vi "__2400_init.vi"(4 "‚SW":bool=TRUE, 5 "volt_range(mV)":dbl, 6 "curr_range(mA)":dbl, 7 "GPIB":string="24") -> (0 "error out":errorcluster caption="エラー出力")   [LabVIEW 2017]
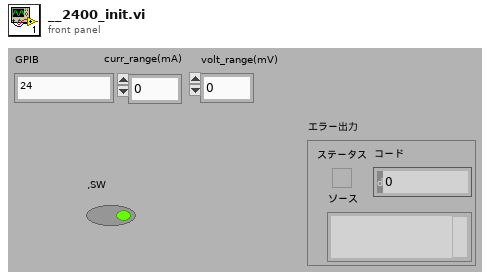
[diagram p1: front panel]
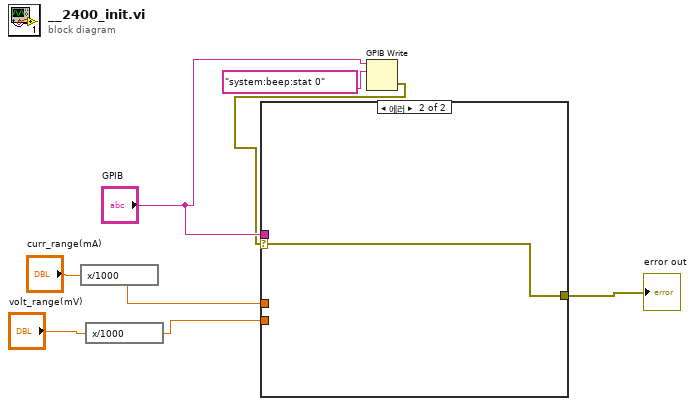
[diagram p0: block diagram]
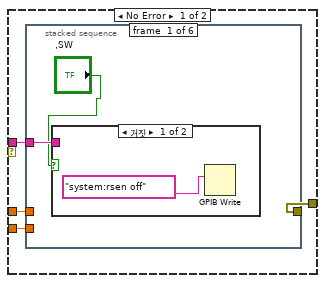
[diagram p2: hidden frame]
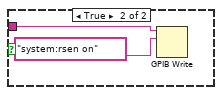
[diagram p3: hidden frame]
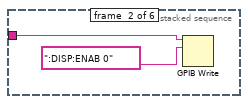
[diagram p4: hidden frame]
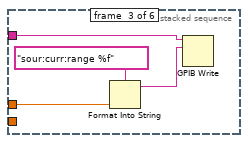
[diagram p5: hidden frame]
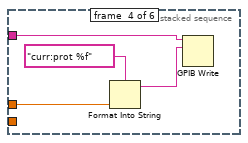
[diagram p6: hidden frame]
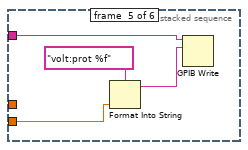
[diagram p7: hidden frame]
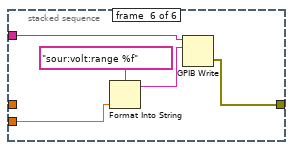
[diagram p8: hidden frame]
diagram:
  n1 = expression code="x/1000"("curr_range(mA)") -> (w7:dbl)
  n2 = expression code="x/1000"("volt_range(mV)") -> (w5:dbl)
  n3 = GPIB Write(0:"GPIB", 1:"system:beep:stat 0") -> (6:w1:errorcluster)  [unwired: 3 in, 1 out]
  n4 = case shown="에러" w1 {
    selector: w1 -> [_ w37]
    tunnel: w7 -> [w12 _]
    tunnel: w5 -> [w11 _]
    tunnel: [w10 w37] -> w4
    tunnel: "GPIB" -> [w9 _]
    frame No Error {
      n5 = stacked-sequence {
        tunnel: w9 -> [w14 w19 w23 w27 w31 w36]
        tunnel: w12 -> [_ _ w22 w25 _ _]
        tunnel: w11 -> [_ _ _ _ w28 w33]
        tunnel: [_ _ _ _ _ w32] -> w10
        frame #0 {
          n6 = case shown="거짓" "‚SW" {
            tunnel: w14 -> [_ w17]
            frame False {
              n7 = GPIB Write(1:"system:rsen off") -> ()  [unwired: 4 in, 2 out]
            }
            frame True {
              n8 = GPIB Write(0:w17, 1:"system:rsen on") -> ()  [unwired: 3 in, 2 out]
            }
          }
        }
        frame #1 {
          n9 = GPIB Write(0:w19, 1:":DISP:ENAB 0") -> ()  [unwired: 3 in, 2 out]
        }
        frame #2 {
          n10 = Format Into String(format string="sour:curr:range %f", w22) -> (resulting string=w21:string)  [unwired: 2 in, 1 out]
          n11 = GPIB Write(0:w23, 1:w21) -> ()  [unwired: 3 in, 2 out]
        }
        frame #3 {
          n12 = Format Into String(format string="curr:prot %f", w25) -> (resulting string=w24:string)  [unwired: 2 in, 1 out]
          n13 = GPIB Write(0:w27, 1:w24) -> ()  [unwired: 3 in, 2 out]
        }
        frame #4 {
          n14 = Format Into String(format string="volt:prot %f", w28) -> (resulting string=w29:string)  [unwired: 2 in, 1 out]
          n15 = GPIB Write(0:w31, 1:w29) -> ()  [unwired: 3 in, 2 out]
        }
        frame #5 {
          n16 = Format Into String(format string="sour:volt:range %f", w33) -> (resulting string=w34:string)  [unwired: 2 in, 1 out]
          n17 = GPIB Write(0:w36, 1:w34) -> (6:w32:errorcluster)  [unwired: 3 in, 1 out]
        }
      }
    }
    frame Error {
    }
  }
  "error out" <- w4
